vi "Uart Set Parameters.vi"(5 "Stop Bits":u8, 6 "Parity":T1(ring), 7 "Data Bits":u8, 8 "error in (no error)":errorcluster, 9 "Baudrate":u32, 10 "Channel":u8, 11 "LMH_LINX in":refnum<class "LINX API.lvclass">) -> (0 "error out":errorcluster, 1 "Actual Baudrate":u32, 3 "LMH_LINX out":refnum<class "LINX API.lvclass">)   [LabVIEW 2020, in "LINX API.lvclass"]
uses:
  LINX API.lvclass
  LINX API.lvclass/LINX API.ctl
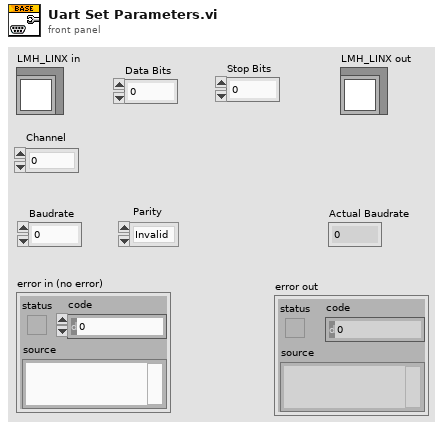
[diagram p1: front panel]
types:
  T1 = enum8{"Invalid", "None", "Odd", "Even", "Mark", "Space"}
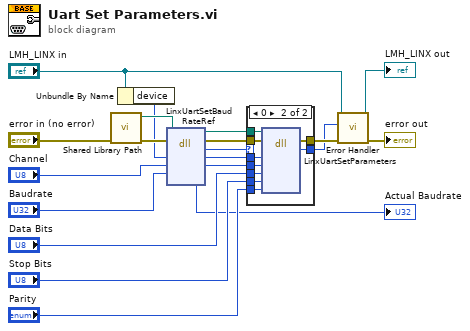
[diagram p0: block diagram]
diagram:
  n1 = call "Shared Library Path.vi"("error in (no error)"="error in (no error)") -> ("error out"=w11:errorcluster, "Path"=w8:path)  [unwired: 9 out]
  n2 = Unbundle By Name("LMH_LINX in") -> ("device"=w4:u64)
  n3 = dll-call lib="Z:/Development/LabVIEW Hobbyist Toolkit/LabVIEW/vi.lib/MakerHub/LINX/Resources/libLinxDevice.dll" fn="LinxUartSetBaudRateRef"(path in=w8, error in=w11, "device"=w4, "channel"="Channel", "baudrate"="Baudrate") -> (path out=w7:path, error out=w6:errorcluster, "status"=w1:i32, "device"=w9:u64, "channel"=w10:u8, "actualBaud"=→"Actual Baudrate":u32)  [unwired: 2 in, 1 out]
  n4 = case shown="0" w1 {
    selector: w1 -> [w21 _]
    tunnel: [w22 w31] -> w16
    tunnel: "Data Bits" -> [_ w30]
    tunnel: "Stop Bits" -> [_ w29]
    tunnel: "Parity" -> [_ w28]
    tunnel: [w21 w27] -> w12
    tunnel: w10 -> [_ w26]
    tunnel: w9 -> [_ w25]
    tunnel: w7 -> [_ w24]
    tunnel: w6 -> [w22 w23]
    frame Default {
    }
    frame 0 {
      n5 = dll-call lib="Z:/Development/LabVIEW Hobbyist Toolkit/LabVIEW/vi.lib/MakerHub/LINX/Resources/libLinxDevice.dll" fn="LinxUartSetParameters"(path in=w24, error in=w23, "device"=w25, "channel"=w26, "dataBits"=w30, "stopBits"=w29, "parity"=w28) -> (error out=w31:errorcluster, "status"=w27:i32)  [unwired: 5 in, 2 out]
    }
  }
  n6 = call "Error Handler.vi"("error in (no error)"=w16, "LINX error code"=w12, "LINX Device"="LMH_LINX in") -> ("error out"=→"error out":errorcluster, "LINX Device out"=→"LMH_LINX out":refnum<class "LINX API.lvclass">)  [unwired: 7 out]
